vi "Cockpit MS.vi"(6 "PID Cluster":T3={"L1 to L4 PID Cluster"={"L1 PID Gains"={"Kp"=0.005, "Kd"=0.5, "Ki"=0.0005}, "L2 PID Gains"={"Kp"=0.01, "Kd"=1.0, "Ki"=0.005}, "L3 PID Gains"={"Kp"=0.05, "Kd"=1.0, "Ki"=0.0005}, "L4 PID Gains"={"Kp"=0.1, "Kd"=0.1, "Ki"=0.0005}}, "Stage PID Cluster"={"Stage Z PID"={"Kp"=0.0005, "Kd"=0.001, "Ki"=0.0}, "Stage Y PID"={"Kp"=0.0003, "Kd"=0.01, "Ki"=0.0}, "Stage X PID"={"Kp"=0.0003, "Kd"=0.01, "Ki"=0.0}}, "OCT Z PID Gains"={"Kp"=0.0003, "Kd"=0.0001, "Ki"=0.01}}, 8 "error in":errorcluster, 9 "Offset Home 2 RCM":dbl[](array[numeric])=[0.0, 0.0, 0.0, 0.0], 10 "Prev Posit Cluster":T2={"Prev L1 to L4 Posit"=[-0.5319, -0.035669172703475985, -2.0566170657346783, 0.9099264705882353], "Prev Stage Posit"=[6.002553885707208, 5.996566124542428, 5.995469940427586], "Prev OCT Z Posit"=-0.0}, 11 "FPGA VI Reference In":refnum<k20>) -> (0 "error out":errorcluster, 2 "Last Posit Cluster":T1={"Last L1 to L4 Posit"=[0.0, 0.0, 0.0, 0.0], "Last Stage Posit"=[6.0, 6.0, 6.0], "Last OCT Z Posit"=0.0}, 3 "FPGA VI Reference Out":refnum<k20>)   [LabVIEW 2010]
uses:
  Global Variables.vi
  <vilib>/Platform/TimedLoop/XDataNode/wakeup.ctl
  <vilib>/Platform/TimedLoop/XDataNode/XDNodeRunTimeDep.lvlib
  <vilib>/Platform/TimedLoop/XDataNode/nitl_modes.ctl
  <vilib>/Platform/TimedLoop/XDataNode/timing_clust.ctl
  <vilib>/platform/TimedLoop/XDataNode/XDataNode.xnode
  <vilib>/rvi/interface/nirviReadWriteControl/nirviReadWriteControl.xnode
  Library/KevinLibraryAll/labview/KevLib01.lvlib
  FPGA Bitfiles/IRISSControl_FPGATarget_IRISSFPGAIOv3.3_r-h2UkgnQFc.lvbitx
  IRISS_FPGA_IO_v3.3.vi
panel:
  out "Pincer Cmd":sgl
  out "L1 to L4 Posit":dbl[](array[numeric])
  out "L1 to L4 Remote cmd":sgl[](array[numeric])
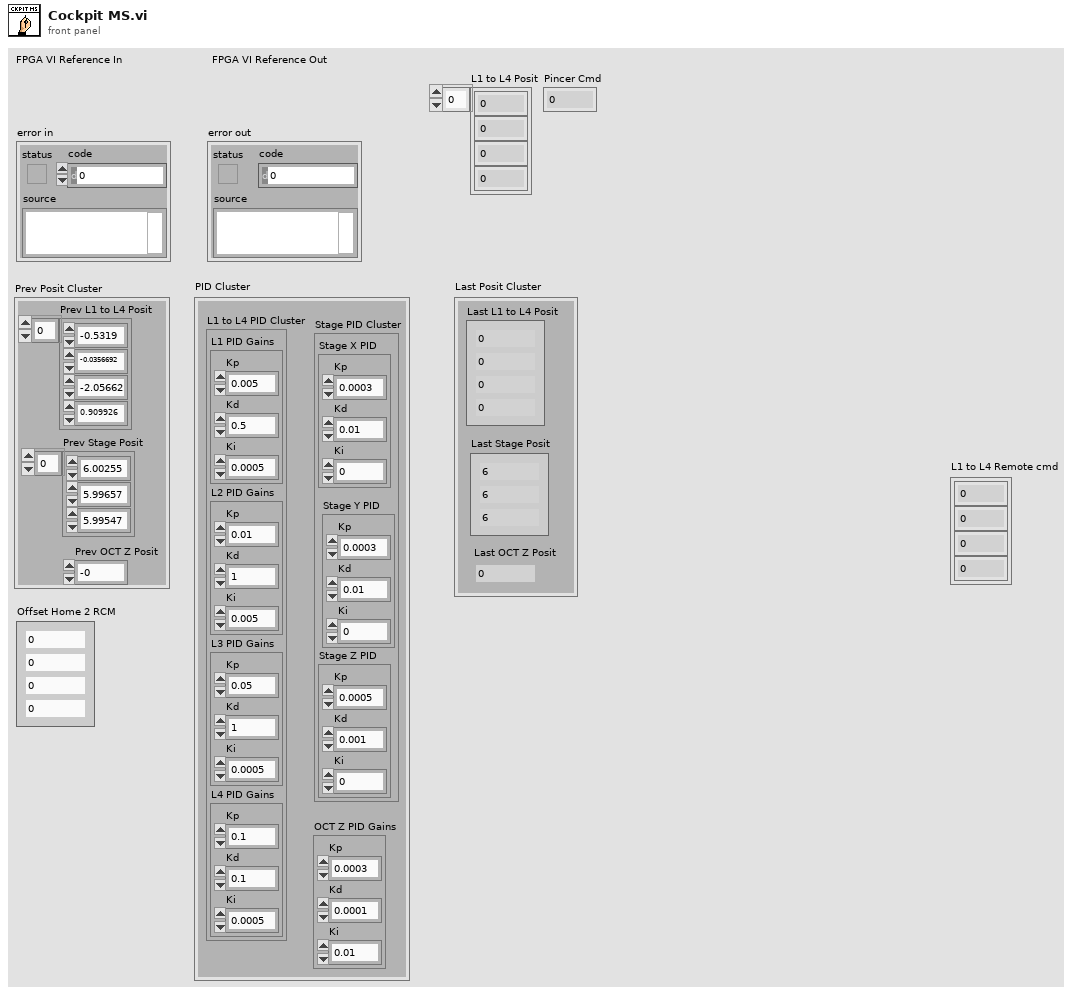
[diagram p1: front panel]
types:
  T1 = cluster{"Last L1 to L4 Posit":dbl[], "Last Stage Posit":dbl[], "Last OCT Z Posit":dbl}
  T2 = cluster{"Prev L1 to L4 Posit":dbl[], "Prev Stage Posit":dbl[], "Prev OCT Z Posit":dbl}
  T3 = cluster{"L1 to L4 PID Cluster":cluster{"L1 PID Gains":cluster{"Kp":dbl, "Kd":dbl, "Ki":dbl}, "L2 PID Gains":cluster{"Kp":dbl, "Kd":dbl, "Ki":dbl}, "L3 PID Gains":cluster{"Kp":dbl, "Kd":dbl, "Ki":dbl}, "L4 PID Gains":cluster{"Kp":dbl, "Kd":dbl, "Ki":dbl}}, "Stage PID Cluster":cluster{"Stage Z PID":cluster{"Kp":dbl, "Kd":dbl, "Ki":dbl}, "Stage Y PID":cluster{"Kp":dbl, "Kd":dbl, "Ki":dbl}, "Stage X PID":cluster{"Kp":dbl, "Kd":dbl, "Ki":dbl}}, "OCT Z PID Gains":cluster{"Kp":dbl, "Kd":dbl, "Ki":dbl}}
  T4 = typedef "XDNodeRunTimeDep.lvlib/timing_clust.ctl" = cluster{"Expected End [f-1]":u64, "Actual End [f-1]":u64, "Finished Late? [f-1]":bool, "Expected End [i-1]":u64, "Actual End [i-1]":u64, "Finished Late? [i-1]":bool, "Expected Start [i]":u64, "Actual Start [i]":u64, "Expected Start [f]":u64, "Actual Start [f]":u64, "Source Name":string, "Structure Name":string, "Period":i64, "Deadline":i64, "Offset":i64, "Start":i64, "Priority":i32, "Timeout":i32, "Mode":T5, "Wakeup Reason":T6, "Error":errorcluster, "Source Type":string, "Secondary Source Type":string, "Global End Time":u64, "Global Start Time":u64, "Frame Duration":u64, "Iteration Duration":u64, "Assigned CPU":i32, "I/O Scan Engine Mode":u32}
  T5 = typedef "XDNodeRunTimeDep.lvlib/nitl_modes.ctl" = enum32{"No Change", "Process missed periods, maintain original phase", "Discard missed periods, maintain original phase", "Process missed periods, ignore original phase", "Discard missed periods, ignore original phase"}
  T6 = typedef "XDNodeRunTimeDep.lvlib/wakeup.ctl" = enum32{"Normal", "Aborted", "Asynchronous wakeup", "Timing source error", "Timed loop error", "Timeout"}
  T7 = cluster{"Stop Vacuum":bool, "Vacuum Force":i8, "Max Limit [mmHg]":dbl, "Slide in":i8, "Irrigation?":bool}
  T8 = cluster{"L1 PID Gains":cluster{"Kp":dbl, "Kd":dbl, "Ki":dbl}, "L2 PID Gains":cluster{"Kp":dbl, "Kd":dbl, "Ki":dbl}, "L3 PID Gains":cluster{"Kp":dbl, "Kd":dbl, "Ki":dbl}, "L4 PID Gains":cluster{"Kp":dbl, "Kd":dbl, "Ki":dbl}}
  T9 = cluster{"Stage Z PID":cluster{"Kp":dbl, "Kd":dbl, "Ki":dbl}, "Stage Y PID":cluster{"Kp":dbl, "Kd":dbl, "Ki":dbl}, "Stage X PID":cluster{"Kp":dbl, "Kd":dbl, "Ki":dbl}}
  T10 = cluster{"Accurus button":bool[], "Accurus engaged?":bool, "Vacuum Force":i32, "Accurus Ch. A Vout":dbl, "Accurus Ch. B Vout":dbl, "Irrigation engaged?":bool}
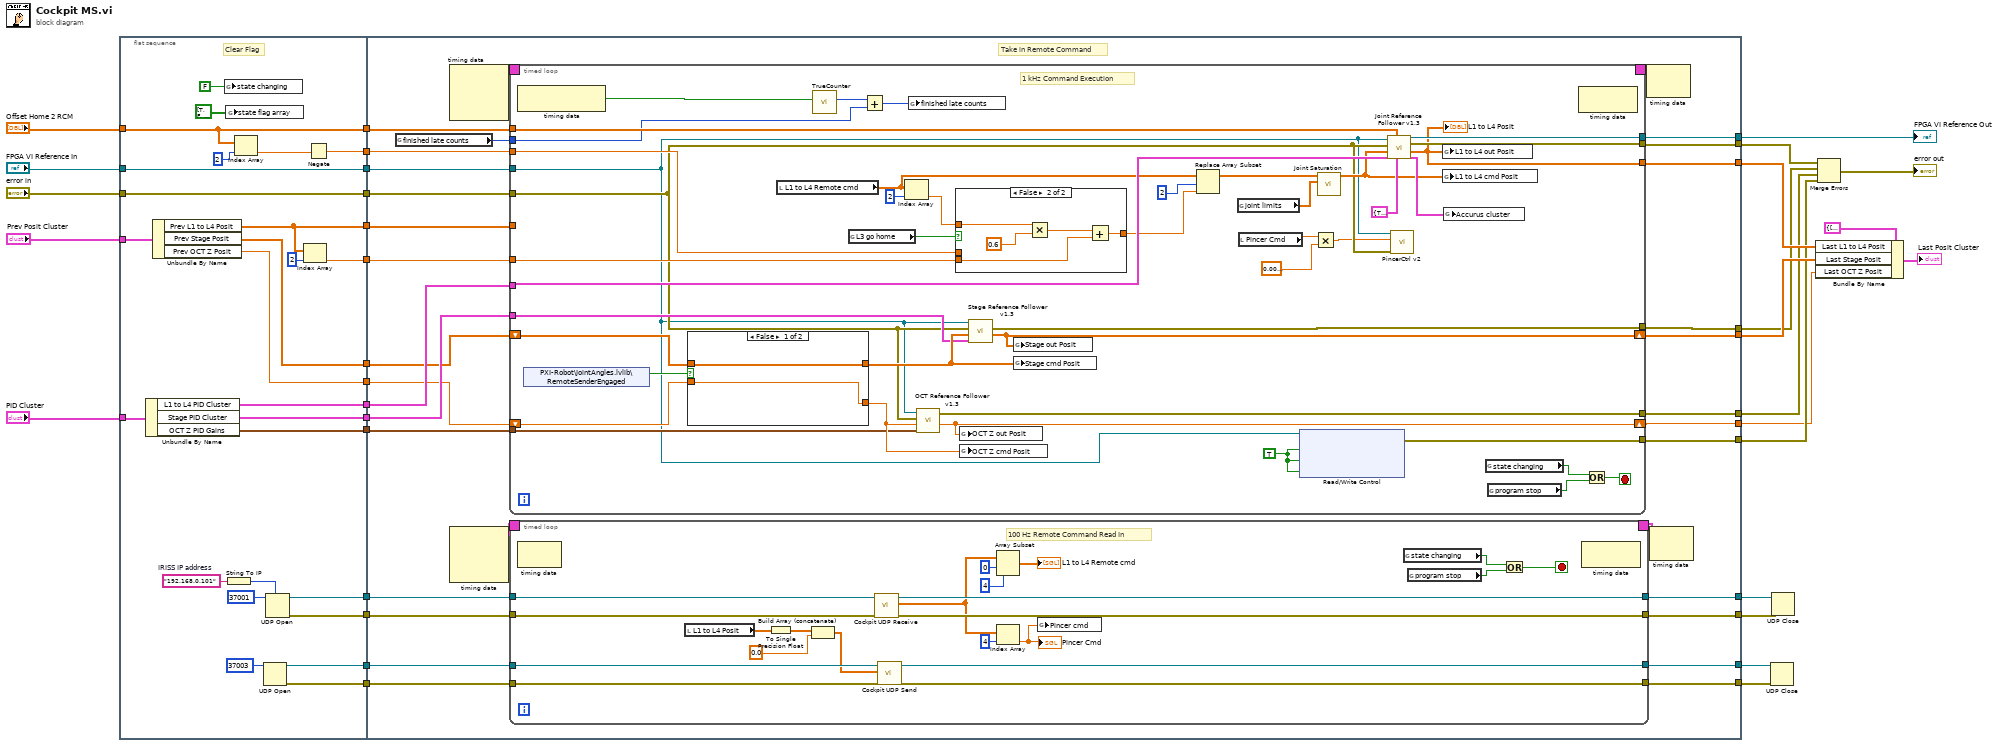
[diagram p0: block diagram]
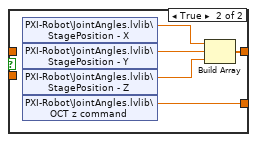
[diagram p2: hidden frame]
diagram:
  n1 = flat-sequence {
    tunnel: [w40] -> w35
    tunnel: [w58] -> w34
    tunnel: "FPGA VI Reference In" -> [w58]
    tunnel: [w57] -> w32
    tunnel: "error in" -> [w57]
    tunnel: [w50] -> w30
    tunnel: "Offset Home 2 RCM" -> [w50]
    tunnel: "Prev Posit Cluster" -> [w45]
    tunnel: [w55] -> w27
    tunnel: "PID Cluster" -> [w54]
    tunnel: [w53] -> w25
    tunnel: [w52] -> w24
    tunnel: [w48] -> w23
    tunnel: [w47] -> w11
    tunnel: [w46] -> w10
    tunnel: [w44] -> w9
    tunnel: [w43] -> w8
    tunnel: [w38] -> w7
    tunnel: [w37] -> w6
    tunnel: [w36] -> w5
    tunnel: w35 -> [w89]
    tunnel: w34 -> [w88]
    tunnel: w32 -> [w87]
    tunnel: w30 -> [w86]
    tunnel: w27 -> [w85]
    tunnel: w25 -> [w84]
    tunnel: w24 -> [w83]
    tunnel: w23 -> [w82]
    tunnel: [w81] -> w13
    tunnel: [w80] -> w19
    tunnel: [w79] -> w20
    tunnel: [w69] -> w17
    tunnel: [w70] -> w16
    tunnel: [w78] -> w14
    tunnel: [w77] -> w15
    tunnel: [w71] -> w12
    tunnel: w11 -> [w76]
    tunnel: w10 -> [w75]
    tunnel: w9 -> [w73]
    tunnel: w8 -> [w72]
    tunnel: w7 -> [w68]
    tunnel: w6 -> [w67]
    tunnel: w5 -> [w66]
    tunnel: [w65] -> w4
    tunnel: [w64] -> w3
    tunnel: [w63] -> w2
    tunnel: [w62] -> w1
    frame #0 {
      w42 = "192.168.0.101"  # IRISS IP address
      # "Clear Flag"
      n2 = Unbundle By Name(w54) -> ("L1 to L4 PID Cluster"=w53:T8, "Stage PID Cluster"=w47:T9, "OCT Z PID Gains"=w46:cluster{"Kp":dbl, "Kd":dbl, "Ki":dbl})
      n3 = Unbundle By Name(w45) -> ("Prev L1 to L4 Posit"=w55:dbl[], "Prev Stage Posit"=w44:dbl[], "Prev OCT Z Posit"=w43:dbl)
      n4 = global write "Global Variables.vi" "state changing"(FALSE ("state changing")) -> ()
      n5 = global write "Global Variables.vi" "state flag array"(bool[] [TRUE, FALSE, FALSE, FALSE, FALSE, FALSE, FALSE, FALSE, FALSE] ("state flag array")) -> ()
      n6 = String To IP(1:w42) -> (0:w41:u32)
      n7 = Index Array(array=w50, index=2) -> (element=w49:dbl)
      n8 = UDP Open(11:u16 37003 ("port")) -> (port=w37:refnum<k16>, 0:w36:errorcluster)  [unwired: 4 in, 1 out]
      n9 = UDP Open(7:w41, 11:u16 37001 ("port")) -> (port=w40:refnum<k16>, 0:w38:errorcluster)  [unwired: 3 in, 1 out]
      n10 = Index Array(array=w55, index=2) -> (element=w52:dbl)
      n11 = Negate(x=w49) -> (-x=w48:dbl)
    }
    frame #1 {
      # "Take in Remote Command"
      n12 = global read "Global Variables.vi" "finished late counts"() -> (w74:u16)
      n13 = node-c288() -> (w93:T4)  [unwired: 3 in]
      n14 = node-c288() -> (w91:T4)  [unwired: 3 in]
      n15 = timed-loop {
        timing: w93 -> [_]
        timing-out: [_] -> w92
        tunnel: w88 -> [w122]
        tunnel: w87 -> [w123]
        tunnel: w86 -> [w156]
        tunnel: w85 -> [_]
        tunnel: w84 -> [w153]
        tunnel: w83 -> [w152]
        tunnel: w82 -> [w149]
        tunnel: [w148] -> w81
        tunnel: [w147] -> w80
        tunnel: [w146] -> w79
        tunnel: [w145] -> w78
        tunnel: [w144] -> w77
        tunnel: w76 -> [w142]
        tunnel: w75 -> [w141]
        tunnel: w74 -> [w137]
        shift-right: [w133] -> w70
        shift-left: w73 -> [w136]
        shift-right: [w134] -> w71
        shift-left: w72 -> [w135]
        tunnel: [w130] -> w69
        stop <- w161 stop-if-true
        w129 = TRUE ("Conn0/DIO15 Button 4")
        # "1 kHz Command Execution"
        n16 = node-c288() -> (w140:bool)  [unwired: 1 in]
        n17 = shared-variable "PXI-Robot\\JointAngles.lvlib\\RemoteSenderEngaged"() -> (w132:bool)  [unwired: 1 in, 1 out]
        n18 = case shown="False" w132 {
          tunnel: [w163 w168] -> w155
          tunnel: [w162 w164] -> w154
          tunnel: w136 -> [w163 _]
          tunnel: w135 -> [w162 _]
          frame False {
          }
          frame True {
            n19 = shared-variable "PXI-Robot\\JointAngles.lvlib\\StagePosition - X"() -> (w165:dbl)  [unwired: 1 in, 1 out]
            n20 = shared-variable "PXI-Robot\\JointAngles.lvlib\\StagePosition - Y"() -> (w166:dbl)  [unwired: 1 in, 1 out]
            n21 = shared-variable "PXI-Robot\\JointAngles.lvlib\\StagePosition - Z"() -> (w167:dbl)  [unwired: 1 in, 1 out]
            n22 = shared-variable "PXI-Robot\\JointAngles.lvlib\\OCT z command"() -> (w164:dbl)  [unwired: 1 in, 1 out]
            n23 = Build Array(w165, w166, w167) -> (w168:dbl[])
          }
        }
        n24 = local read "L1 to L4 Remote cmd"() -> (w131:sgl[])
        n25 = call "TrueCounter.vi"("True?"=w140) -> ("True Count"=w138:u16)  [unwired: 10 in]
        n26 = global read "Global Variables.vi" "L3 go home"() -> (w159:bool)
        n27 = Add(x=w138, y=w137) -> (x+y=w139:u16)
        n28 = Index Array(array=w131, index=2) -> (element=w157:sgl)
        n29 = global write "Global Variables.vi" "finished late counts"(w139) -> ()
        n30 = call "OCT Reference Follower v1.3.vi"("OCT Z PID Gains"=w141, "OCT  Z cmd Posit [mm]"=w154, "error in"=w123, "FPGA VI Reference In"=w122) -> ("OCT  Z out Posit [mm]"=w134:dbl, "error out"=w145:errorcluster)  [unwired: 5 in, 1 out]
        n31 = case shown="False" w159 {
          tunnel: [w169 w174] -> w150
          tunnel: w157 -> [_ w171]
          tunnel: w152 -> [_ w170]
          tunnel: w149 -> [w169 _]
          frame True {
            # "Go Home"
          }
          frame False {
            # "Scale = 1 : 0.15; cmd = 20 @ RCM"
            n32 = Multiply(x=w171, y=0.6) -> (x*y=w173:dbl)
            n33 = Add(x=w173, y=w170) -> (x+y=w174:dbl)
          }
        }
        n34 = global write "Global Variables.vi" "OCT Z out Posit"(w134) -> ()
        n35 = global write "Global Variables.vi" "OCT Z cmd Posit"(w154) -> ()
        n36 = call "Stage Reference Follower v1.3.vi"("Stage PID Cluster"=w142, "Stage cmd Posit [mm]"=w155, "error in"=w123, "FPGA VI Reference In"=w122) -> ("Stage out Posit [mm]"=w133:dbl[], "error out"=w144:errorcluster)  [unwired: 5 in, 1 out]
        n37 = global write "Global Variables.vi" "Stage out Posit"(w133) -> ()
        n38 = global write "Global Variables.vi" "Stage cmd Posit"(w155) -> ()
        n39 = Replace Array Subset(array=w131, new element=w150, index=2) -> (w125:sgl[])
        n40 = global read "Global Variables.vi" "joint limits"() -> (w127:dbl[][])
        n41 = local read "Pincer Cmd"() -> (w121:sgl)
        n42 = xnode "Read/Write Control"("FPGA VI Reference In"=w122, "Conn0/DIO12 Button 1"=w129, "Conn0/DIO13 Button 2"=w129, "Conn0/DIO15 Button 4"=w129) -> ("error out"=w148:errorcluster)  [unwired: 1 in, 1 out]
        n43 = Multiply(x=w121, y=sgl 0.01) -> (x*y=w120:sgl)
        n44 = call "Joint Saturation.vi"("Joint Bounds [Deg/mm]"=w127, "Ref Array [Deg/mm]"=w125) -> ("Sat Ref Array [Deg/mm]"=w124:dbl[])  [unwired: 9 in]
        n45 = call "Joint Reference Follower v1.3.vi"("Accurus Ctrl Cluster"=T7 {"Stop Vacuum"=TRUE, "Vacuum Force"=0, "Max Limit [mmHg]"=600.0, "Slide in"=0, "Irrigation?"=TRUE}, "Offset Home2RCM [deg/mm]"=w156, "PID Ctrl Cluster"=w153, "Ref Array [deg/mm]"=w124, "error in"=w123, "FPGA VI Reference In"=w122) -> ("Accurus Output Cluster"=w128:T10, "Output Posit Array [deg/mm]"=w130:dbl[], "error out"=w147:errorcluster, "FPGA VI Reference Out"=w146:refnum<k20>)  [unwired: 2 in]
        "L1 to L4 Posit" <- w130
        n46 = call "PincerCtrl v2.vi"("error in"=w123, "Motion [%]"=w120, "FPGA VI Reference In"=w122) -> ()  [unwired: 7 in, 2 out]
        n47 = global write "Global Variables.vi" "L1 to L4 out Posit"(w130) -> ()
        n48 = global write "Global Variables.vi" "L1 to L4 cmd Posit"(w124) -> ()
        n49 = global write "Global Variables.vi" "Accurus cluster"(w128) -> ()
        n50 = global read "Global Variables.vi" "state changing"() -> (w160:bool)
        n51 = global read "Global Variables.vi" "program stop"() -> (w143:bool)
        n52 = node-c288() -> ()  [unwired: 1 in, 1 out]
        n53 = Or(x=w160, y=w143) -> (x .or. y?=w161:bool)
      }
      n54 = timed-loop {
        timing: w91 -> [_]
        timing-out: [_] -> w90
        tunnel: w89 -> [w111]
        tunnel: w68 -> [w110]
        tunnel: w67 -> [w109]
        tunnel: w66 -> [w108]
        tunnel: [w105] -> w65
        tunnel: [w104] -> w64
        tunnel: [w99] -> w63
        tunnel: [w98] -> w62
        stop <- w114 stop-if-true
        # "100 Hz Remote Command Read In"
        n55 = node-c288() -> ()  [unwired: 1 in, 1 out]
        n56 = local read "L1 to L4 Posit"() -> (w103:dbl[])
        n57 = To Single Precision Float(number=w103) -> (single precision float=w102:sgl[])
        n58 = Build Array (concatenate)(w102, sgl 0.0 ("y")) -> (w100:sgl[])
        n59 = call "Cockpit UDP Receive.vi"("error in"=w110, "connection ID"=w111) -> ("error out"=w104:errorcluster, "read UDP array"=w96:sgl[], "connection ID out"=w105:refnum<k16>)  [unwired: 7 in]
        n60 = call "Cockpit UDP Send.vi"("error in"=w108, "write UDP array"=w100, "connection ID"=w109) -> ("error out"=w98:errorcluster, "connection ID out"=w99:refnum<k16>)  [unwired: 7 in]
        n61 = Array Subset(array=w96, index=0, length=4) -> (→"L1 to L4 Remote cmd":sgl[])
        n62 = Index Array(array=w96, index=4) -> (element=w94:sgl)
        "Pincer Cmd" <- w94
        n63 = global write "Global Variables.vi" "Pincer cmd"(w94) -> ()
        n64 = global read "Global Variables.vi" "state changing"() -> (w113:bool)
        n65 = global read "Global Variables.vi" "program stop"() -> (w112:bool)
        n66 = Or(x=w113, y=w112) -> (x .or. y?=w114:bool)
        n67 = node-c288() -> ()  [unwired: 1 in, 1 out]
      }
      n68 = node-c288(w92) -> ()  [unwired: 1 out]
      n69 = node-c288(w90) -> ()  [unwired: 1 out]
    }
  }
  n70 = UDP Close(connection ID=w2, 8:w1) -> ()  [unwired: 2 out]
  n71 = UDP Close(connection ID=w4, 8:w3) -> ()  [unwired: 2 out]
  n72 = Bundle By Name(cluster=T1 {"Last L1 to L4 Posit"=[-0.5607, -0.038216970753724266, -2.0806193533568895, 1.1787683823529411], "Last Stage Posit"=[6.002553885707208, 5.996566124542428, 5.995469940427586], "Last OCT Z Posit"=-0.0} ("Last Posit Cluster 2"), "Last L1 to L4 Posit"=w17, "Last Stage Posit"=w16, "Last OCT Z Posit"=w12) -> (→"Last Posit Cluster":T1)
  n73 = Merge Errors(w19, w15, w14, w13) -> (→"error out":errorcluster)
  "FPGA VI Reference Out" <- w20
